vi "Face Recognition with Point Following.vi"() -> ()   [LabVIEW 2014]
doc: "This example shows how to use the Lucas Kanade Pyramid motion estimation VI to track features in a sequence of images in NI Vision. The VI reads the frames from an AVI file and tracks user specified features in the image from frame to frame."
uses:
  <vilib>/userdefined/High Color/IMAQdx.ctl
  <vilib>/vision/driver/NI_Vision_Acquisition_Software.lvlib
  <vilib>/vision/NI_Vision_Development_Module.lvlib
panel:
  out "Face Found":bool
  in  "Show Templates":bool=TRUE
  out "Preview":T1(plugin-control)
  in  "Lip Min Score":sgl=700.0
  in  "Nose Min Score":sgl=700.0
  in  "Eye Min Score":sgl=700.0
  out "Lips Template":T1(plugin-control)
  out "Nose Template":T1(plugin-control)
  out "Eye Template":T1(plugin-control)
  in  "Options":T2={"Level"=4, "maxiteration"=20, "windowsize"=20, "threshold"=1.0}
  in  "Stop":bool
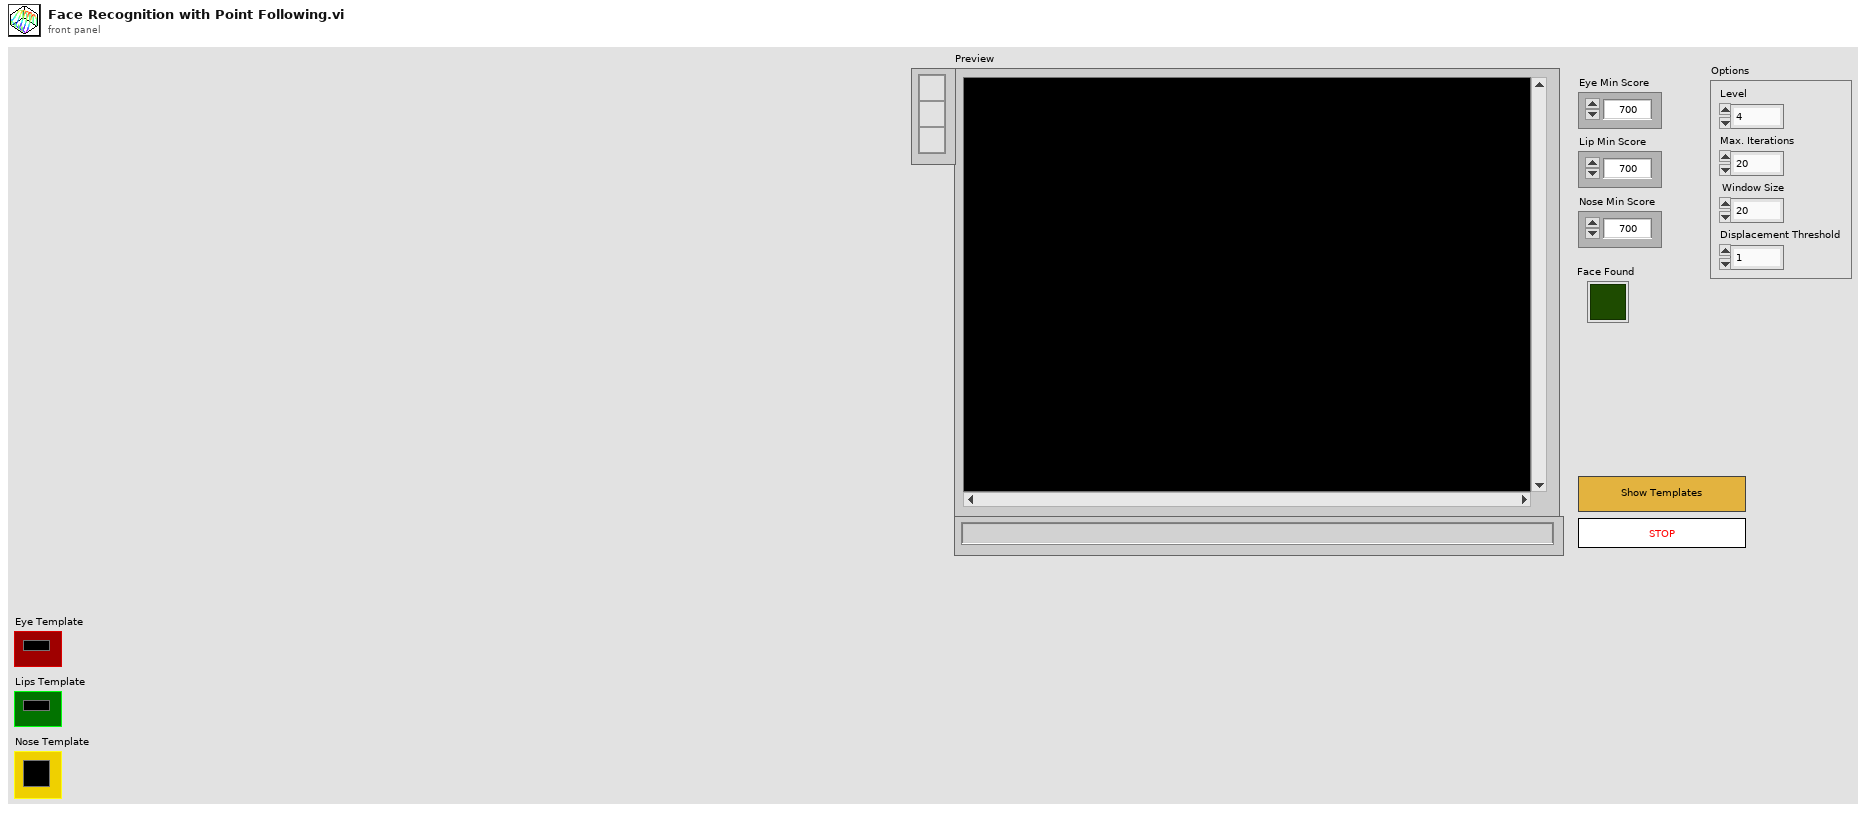
[diagram p1: front panel]
types:
  T1 = typedef "IMAQ Image.ctl" = refnum<image>
  T2 = cluster{"Level":i32, "maxiteration":i32, "windowsize":i32, "threshold":dbl}
  T3 = typedef "Image Type" = u32
  T4 = typedef "IMAQdx.ctl" = refnum<k21>
  T5 = cluster{"Position":cluster{"x":sgl, "y":sgl}, "Angle":sgl, "Scale":sgl, "Score":sgl, "Bounding Box":cluster{"x":sgl, "y":sgl}[]}[]
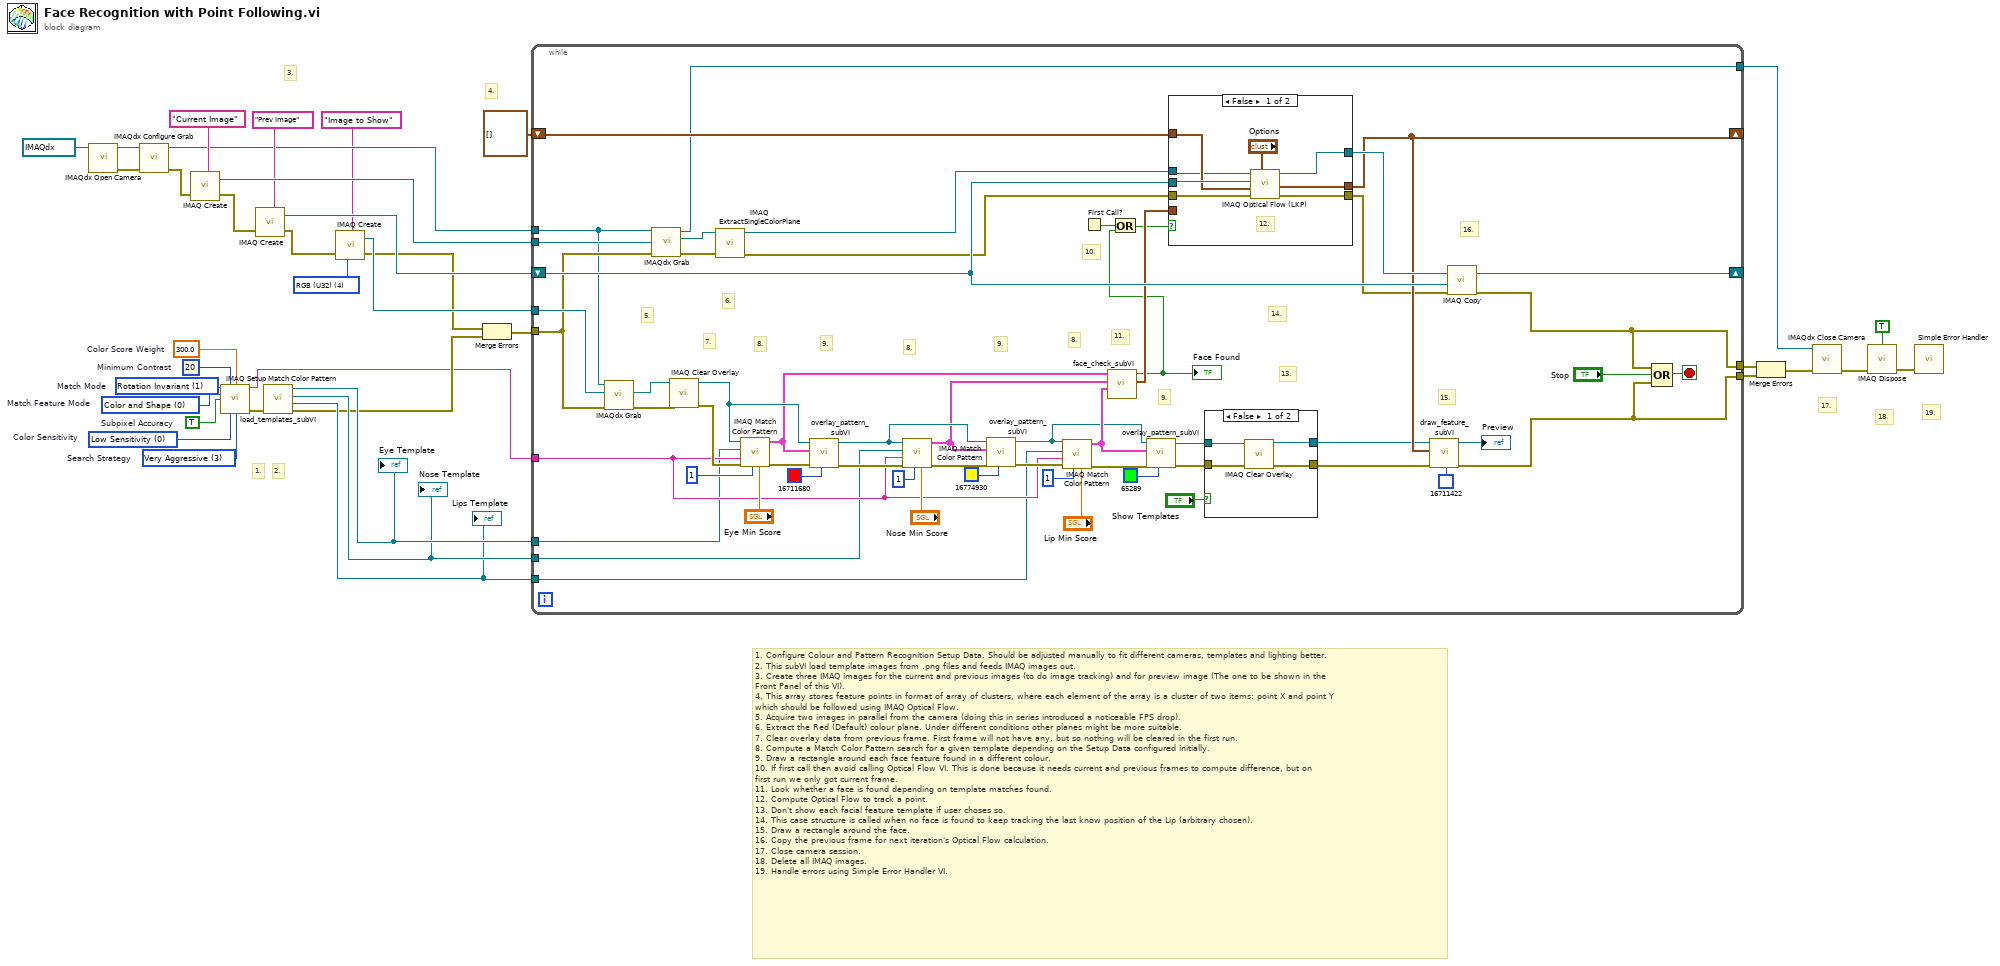
[diagram p0: block diagram]
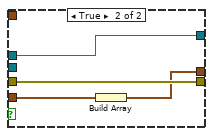
[diagram p3: hidden frame]
diagram:
  w17 = T3 4 items=["Grayscale (U8)", "Grayscale (I16)", "Grayscale (SGL)", "Complex (CSG)", "RGB (U32)", "HSL (U32)", "RGB (U64)", "Grayscale (U16)"] ("Image Type")
  w21 = TRUE  # Subpixel Accuracy
  w27 = u32 0 items=["Color and Shape", "Color", "Shape"]  # Match Feature Mode
  w26 = u32 3 items=["Conservative", "Balance", "Aggressive", "Very Aggressive"]  # Search Strategy
  w25 = 20  # Minimum Contrast
  w24 = sgl 300.0  # Color Score Weight
  w23 = u32 0 items=["Low Sensitivity", "Medium Sensitivity", "High Sensitivity"]  # Color Sensitivity
  w22 = u32 1 items=["Shift Invariant", "Rotation Invariant"]  # Match Mode
  # "1. Configure Colour and Pattern Recognition Setup Data. Should be adjusted manually to fit different cameras, templates and lighting better.\n2. This subVI load template images from .png files and feeds IMAQ images out.\n3. Create three IMAQ images for the current and previous images (to do image tracking) and for preview image (The one to be shown in the\nFront Panel of this VI).\n4. This array stores feature points in format of array of clusters, where each element of the array is a cluster of two items: point X and point Y \nwhich should be followed using IMAQ Optical Flow.\n5. Acquire two images in parallel from the camera (doing this in series introduced a noticeable FPS drop).\n6. Extract the Red (Default) colour plane. Under different conditions other planes might be more suitable.\n7. Clear overlay data from previous frame. First frame will not have any, but so nothing will be cleared in the first run.\n8. Compute a Match Color Pattern search for a given template depending on the Setup Data configured initially.\n9. Draw a rectangle around each face feature found in a different colour.\n10. If first call then avoid calling Optical Flow VI. This is done because it needs current and previous frames to compute difference, but on\nfirst run we only got current frame.\n11. Look whether a face is found depending on template matches found.\n12. Compute Optical Flow to track a point.\n13. Don't show each facial feature template if user choses so.\n14. This case structure is called when no face is found to keep tracking the last know position of the Lip (arbitrary chosen).\n15. Draw a rectangle around the face.\n16. Copy the previous frame for next iteration's Optical Flow calculation.\n17. Close camera session.\n18. Delete all IMAQ images.\n19. Handle errors using Simple Error Handler VI."
  # "19."
  # "17."
  # "4."
  # "3."
  # "3."
  # "3."
  # "2."
  # "1."
  # "18."
  n1 = call <vilib>:"IMAQdx Open Camera.vi"("Session In"=T4 "cam0") -> ("error out"=w31:errorcluster, "Session Out"=w32:T4)  [unwired: 9 in]
  n2 = call <vilib>:"IMAQdx Configure Grab.vi"("error in"=w31, "Session In"=w32) -> ("error out"=w10:errorcluster, "Session Out"=w28:T4)  [unwired: 8 in]
  n3 = call "IMAQ Create"("Image Name"="Current Image", "error in (no error)"=w10) -> ("New Image"=w36:T1, "error out"=w9:errorcluster)  [unwired: 2 in, 1 out]
  n4 = call "IMAQ Setup Match Color Pattern"("Match Mode"=w22, "Minimum Contrast"=w25, "Color Score Weight"=w24, "Match Feature Mode"=w27, "Subpixel Accuracy"=w21, "Color Sensitivity"=w23, "Search Strategy"=w26) -> ("Match Color Pattern Setup Data"=w4:string, "error out"=w20:errorcluster)  [unwired: 7 in]
  n5 = call "IMAQ Create"("Image Name"="Prev Image", "error in (no error)"=w9) -> ("New Image"=w29:T1, "error out"=w8:errorcluster)  [unwired: 2 in, 1 out]
  n6 = call "load_templates_subVI.vi"("error in (no error)"=w20) -> ("error out"=w6:errorcluster, "Lips Template"=w14:T1, "Nose Template"=w15:T1, "Eye Template"=w16:T1)  [unwired: 7 in]
  "Eye Template" <- w16
  "Nose Template" <- w15
  "Lips Template" <- w14
  n7 = call "IMAQ Create"("Image Name"="Image to Show", "Image Type"=w17, "error in (no error)"=w8) -> ("New Image"=w18:T1, "error out"=w7:errorcluster)  [unwired: 1 in, 1 out]
  n8 = Merge Errors(w7, w6) -> (w5:errorcluster)
  n9 = while {
    tunnel: w36 -> [w91]
    shift-right: [w93] -> _
    shift-left: w29 -> [w94]
    shift-right: [w54] -> _
    shift-left: cluster{"X":sgl, "Y":sgl}[] [] ("Feature Points Out") -> [w92]
    tunnel: w28 -> [w45]
    tunnel: [w90] -> w34
    tunnel: w4 -> [w63]
    tunnel: w16 -> [w62]
    tunnel: w15 -> [w61]
    tunnel: w14 -> [w60]
    tunnel: w18 -> [w58]
    tunnel: w5 -> [w47]
    tunnel: [w42] -> w3
    tunnel: [w41] -> w2
    stop <- w44 stop-if-true
    # "10."
    # "16."
    # "15."
    # "14."
    # "13."
    # "11."
    # "9."
    # "8."
    # "9."
    # "8."
    # "9."
    # "8."
    # "7."
    # "6."
    # "5."
    # "5."
    n10 = call <vilib>:"IMAQdx Grab.vi"("error in"=w47, "Image In"=w58, "Session In"=w45) -> ("error out"=w57:errorcluster, "Image Out"=w56:T1)  [unwired: 5 in, 2 out]
    n11 = call <vilib>:"IMAQdx Grab.vi"("error in"=w47, "Image In"=w91, "Session In"=w45) -> ("error out"=w87:errorcluster, "Image Out"=w64:T1, "Session Out"=w90:T4)  [unwired: 5 in, 1 out]
    n12 = call "IMAQ Clear Overlay"("error in (no error)"=w57, "Image"=w56) -> ("error out"=w85:errorcluster, "Image Out"=w71:T1)  [unwired: 8 in]
    n13 = call "IMAQ ExtractSingleColorPlane"("error in (no error)"=w87, "Image Src"=w64) -> ("error out"=w89:errorcluster, "Image Dst Out"=w88:T1)  [unwired: 8 in]
    n14 = call "IMAQ Match Color Pattern"("Minimum Match Score"="Eye Min Score", "Number of Matches Requested"=1, "error in (no error)"=w85, "Match Color Pattern Setup Data"=w63, "Template Image"=w62, "Image"=w71) -> ("error out"=w84:errorcluster, "Matches"=w68:T5)  [unwired: 3 in, 1 out]
    n15 = call "overlay_pattern_subVI.vi"("Color"=u32 16711680, "error in"=w84, "Matches"=w68, "Image"=w71) -> ("error out"=w81:errorcluster, "Image Out"=w78:T1)  [unwired: 6 in]
    n16 = call "IMAQ Match Color Pattern"("Minimum Match Score"="Nose Min Score", "Number of Matches Requested"=1, "error in (no error)"=w81, "Match Color Pattern Setup Data"=w63, "Template Image"=w61, "Image"=w78) -> ("error out"=w79:errorcluster, "Matches"=w67:T5)  [unwired: 3 in, 1 out]
    n17 = call "overlay_pattern_subVI.vi"("Color"=u32 16774930, "error in"=w79, "Matches"=w67, "Image"=w78) -> ("error out"=w77:errorcluster, "Image Out"=w65:T1)  [unwired: 6 in]
    n18 = call "IMAQ Match Color Pattern"("Minimum Match Score"="Lip Min Score", "Number of Matches Requested"=1, "error in (no error)"=w77, "Match Color Pattern Setup Data"=w63, "Template Image"=w60, "Image"=w65) -> ("error out"=w76:errorcluster, "Matches"=w66:T5)  [unwired: 3 in, 1 out]
    n19 = First Call?() -> (First Call?: T/F=w38:bool)
    n20 = call "face_check_subVI.vi"("Lips Match"=w66, "Nose Match"=w67, "Eye Match"=w68) -> ("Lip Position"=w59:cluster{"x":sgl, "y":sgl}, "Face Found"=w40:bool)  [unwired: 6 in, 1 out]
    "Face Found" <- w40
    n21 = Or(x=w38, y=w40) -> (x .or. y?=w39:bool)
    n22 = call "overlay_pattern_subVI.vi"("Color"=u32 65289, "error in"=w76, "Matches"=w66, "Image"=w65) -> ("error out"=w50:errorcluster, "Image Out"=w52:T1)  [unwired: 6 in]
    n23 = case shown="False" w39 {
      tunnel: w94 -> [w108 _]
      tunnel: w92 -> [w107 _]
      tunnel: [w106 w109] -> w54
      tunnel: w89 -> [w105 w112]
      tunnel: w88 -> [w101 w111]
      tunnel: [w103 w111] -> w86
      tunnel: [w102 w112] -> w46
      tunnel: w59 -> [_ w110]
      frame False {
        # "12."
        n24 = call "IMAQ Optical Flow (LKP)"("Options"="Options", "error in (no error)"=w105, "Feature Points In"=w107, "Previous Frame"=w108, "Current Frame"=w101) -> ("error out"=w102:errorcluster, "Feature Points Out"=w106:cluster{"X":sgl, "Y":sgl}[], "Current Frame Out (dup)"=w103:T1)  [unwired: 1 in, 3 out]
      }
      frame True {
        n25 = Build Array(w110) -> (w109:cluster{"x":sgl, "y":sgl}[])
      }
    }
    n26 = case shown="False" "Show Templates" {
      tunnel: w52 -> [w98 w100]
      tunnel: [w97 w100] -> w51
      tunnel: w50 -> [w96 w99]
      tunnel: [w95 w99] -> w48
      frame False {
        n27 = call "IMAQ Clear Overlay"("error in (no error)"=w96, "Image"=w98) -> ("error out"=w95:errorcluster, "Image Out"=w97:T1)  [unwired: 8 in]
      }
      frame True {
      }
    }
    n28 = call "draw_feature_subVI.vi"("Color"=u32 16711422, "Error In"=w48, "Feature Ponts"=w54, "Image"=w51) -> ("Error Out"=w41:errorcluster, "Image Out"=→"Preview":T1)  [unwired: 6 out]
    n29 = call "IMAQ Copy"("error in (no error)"=w46, "Image Dst"=w94, "Image Src"=w86) -> ("error out"=w42:errorcluster, "Image Dst Out"=w93:T1)  [unwired: 3 out]
    n30 = Compound Arithmetic op=OR(w42, "Stop", w41) -> (w44:bool)
  }
  n31 = Merge Errors(w3, w2) -> (w1:errorcluster)
  n32 = call <vilib>:"IMAQdx Close Camera.vi"("error in"=w1, "Session In"=w34) -> ("error out"=w13:errorcluster)  [unwired: 9 in]
  n33 = call "IMAQ Dispose"("All Images? (No)"=TRUE, "error in (no error)"=w13) -> ("error out"=w12:errorcluster)  [unwired: 1 in, 3 out]
  n34 = call <vilib>:"Simple Error Handler.vi"("error in (no error)"=w12) -> ()  [unwired: 1 in, 8 out]
